vi "Input_Images.vi"(6 "Dark Image In":T2, 9 "Milsec Wait":u32, 10 "CameraDevRef":T1, 11 "Light Image In":T2) -> (2 "Dark Image Out":T2, 3 "Light Image Out":T2)   [LabVIEW 2011]
uses:
  <vilib>/vision/Image Controls.llb/IMAQ Image.ctl
  <vilib>/Rock Robotics/WPI/Camera/WPI_CameraDevRef.ctl
  <vilib>/Rock Robotics/WPI/Relay/WPI_RelayValue.ctl
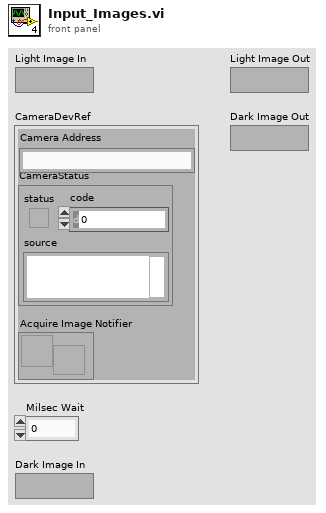
[diagram p1: front panel]
types:
  T1 = typedef "WPI_CameraDevRef.ctl" = cluster{"Camera Address":string, "CameraStatus":errorcluster, "Acquire Image Notifier":refnum<notifier>}
  T2 = typedef "IMAQ Image.ctl" = refnum<image>
  T3 = typedef "WPI_RelayValue.ctl" = enum16{"Off", "On", "Forward", "Reverse"}
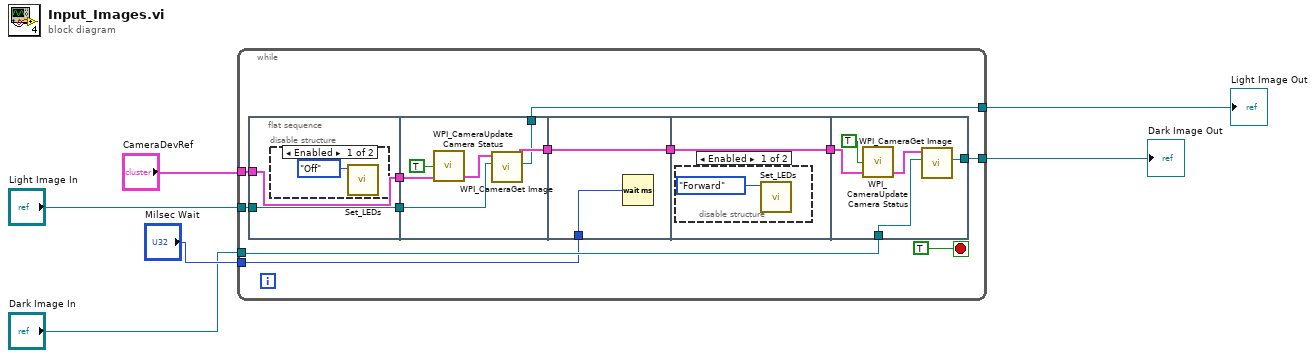
[diagram p0: block diagram]
diagram:
  n1 = while {
    tunnel: "CameraDevRef" -> [w17]
    tunnel: [w16] -> w5
    tunnel: [w13] -> w4
    tunnel: "Light Image In" -> [w14]
    tunnel: "Dark Image In" -> [w9]
    tunnel: "Milsec Wait" -> [w7]
    stop <- TRUE stop-if-true
    n2 = flat-sequence {
      tunnel: w17 -> [w19]
      tunnel: w14 -> [w20]
      tunnel: [w20] -> w12
      tunnel: [w19] -> w11
      tunnel: [w25] -> w15
      tunnel: [w24] -> w13
      tunnel: w12 -> [w23]
      tunnel: w11 -> [w22]
      tunnel: [w29] -> w18
      tunnel: w15 -> [w29]
      tunnel: w7 -> [w28]
      tunnel: w18 -> [w30]
      tunnel: [w30] -> w8
      tunnel: [w32] -> w16
      tunnel: w9 -> [w34]
      tunnel: w8 -> [w33]
      frame #0 {
        n3 = disable-structure shown="Enabled" {
          frame Enabled {
            n4 = call "Set_LEDs.vi"("RelayValue"=WPI_RelayValue."Off") -> ()  [unwired: 10 in, 1 out]
          }
          frame Disabled {
          }
        }
      }
      frame #1 {
        n5 = call <vilib>:"WPI_CameraUpdate Camera Status.vi"("CameraDevRef In"=w22, "Enable Vision"=TRUE) -> ("CameraDevRef Out"=w26:T1)  [unwired: 3 in]
        n6 = call <vilib>:"WPI_CameraGet Image.vi"("Image"=w23, "CameraDevRef"=w26) -> ("Image Out"=w24:T2, "CameraDevRef Out"=w25:T1)  [unwired: 7 in, 1 out]
      }
      frame #2 {
        n7 = Wait (ms)(milliseconds to wait=w28) -> ()  [unwired: 1 out]
      }
      frame #3 {
        n8 = disable-structure shown="Enabled" {
          frame Enabled {
            n9 = call "Set_LEDs.vi"("RelayValue"=WPI_RelayValue."Forward") -> ()  [unwired: 10 in, 1 out]
          }
          frame Disabled {
          }
        }
      }
      frame #4 {
        n10 = call <vilib>:"WPI_CameraUpdate Camera Status.vi"("CameraDevRef In"=w33, "Enable Vision"=TRUE) -> ("CameraDevRef Out"=w36:T1)  [unwired: 3 in]
        n11 = call <vilib>:"WPI_CameraGet Image.vi"("Image"=w34, "CameraDevRef"=w36) -> ("Image Out"=w32:T2)  [unwired: 7 in, 2 out]
      }
    }
  }
  "Dark Image Out" <- w5
  "Light Image Out" <- w4
